vi "StartClone.vi"(7 "ShowPanel? (f)":bool, 8 "error in (no error)":errorcluster, 10 "ModuleName":string="unnamed", 11 "VI Refnum":refnum<vi>) -> (0 "error out":errorcluster, 1 "clBroadcastEvents":T1, 2 "VI Ref":refnum<vi>, 3 "ModuleAdmin":refnum<class "ModuleAdmin.lvclass">)   [LabVIEW 2018, in "FgenShared.lvlib"]
uses:
  FgenShared/FgenShared.lvlib
  FgenShared/clBroadcastEvents.ctl
  FgenShared/clEventType.ctl
  <userlib>/NIST/ModuleAdminLib/ModuleAdmin/ModuleAdmin.lvclass
  C:/Program Files (x86)/National Instruments/LabVIEW 2018/user.lib/NIST/ModuleAdminLib/ModuleAdminBase/ModuleAdminBase.lvclass
  <userlib>/NIST/ModuleAdminLib/CloneRegistration/CloneRegistration.lvclass
  <userlib>/NIST/ModuleAdminLib/ModuleAdmin/ModuleAdmin.lvclass/ModuleAdmin.ctl
  <userlib>/NIST/ModuleAdminLib/ModuleAdmin/Accessors/Write CloneRegRef.vi
  <userlib>/NIST/ModuleAdminLib/ModuleAdmin/Accessors/Write ShowPanel_.vi
  <vilib>/Utility/error.llb/Error Cluster From Error Code.vi
  <vilib>/ErrorRing/Error Ring.xnode
  <userlib>/NIST/ModuleAdminLib/ModuleAdminBase/ModuleAdminBase.lvclass
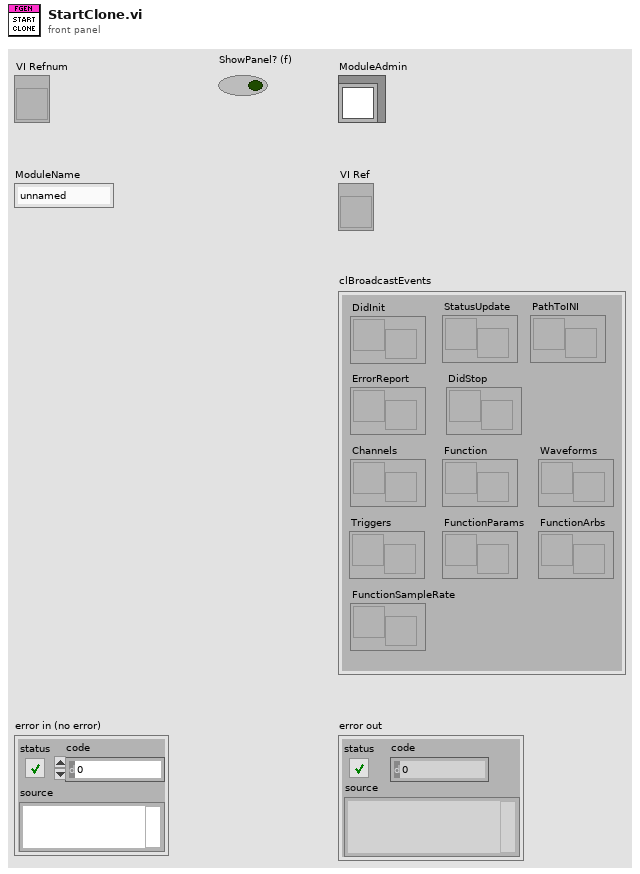
[diagram p1: front panel]
types:
  T1 = typedef "FgenShared.lvlib/clBroadcastEvents.ctl" = cluster{"DidInit":refnum<user-event>, "StatusUpdate":refnum<user-event>, "ErrorReport":refnum<user-event>, "DidStop":refnum<user-event>, "PathToINI":refnum<user-event>, "Channels":refnum<user-event>, "Function":refnum<user-event>, "Waveforms":refnum<user-event>, "Triggers":refnum<user-event>, "FunctionParams":refnum<user-event>, "FunctionArbs":refnum<user-event>, "FunctionSampleRate":refnum<user-event>}
  T2 = enum32{"Bad", "Idle", "Run top level", "Running"}
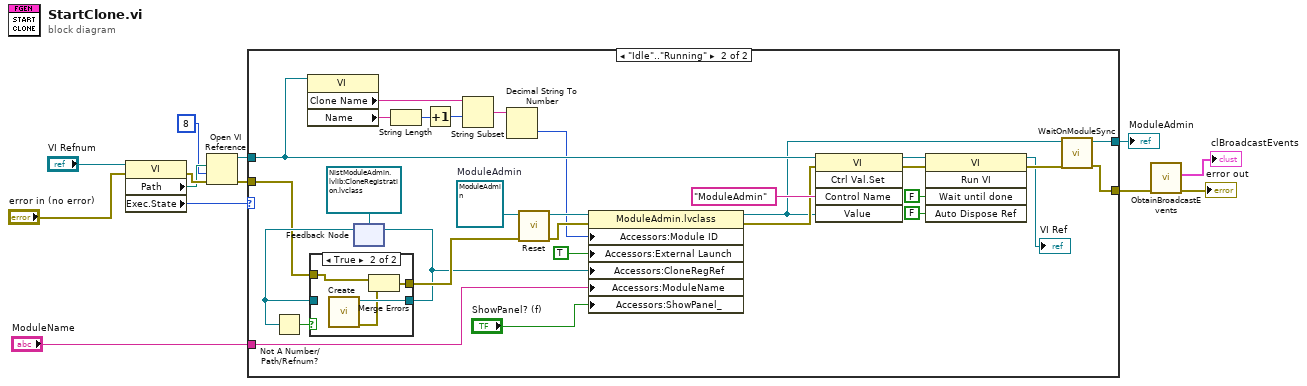
[diagram p0: block diagram]
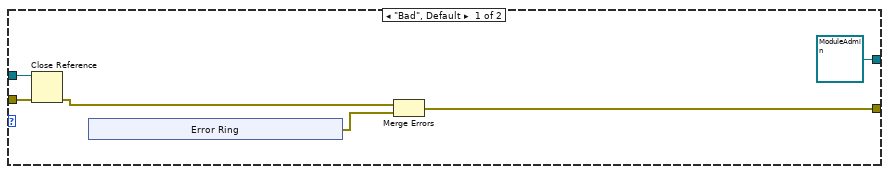
[diagram p2: hidden frame]
diagram:
  n1 = property class="VI"(reference="VI Refnum", error in="error in (no error)") -> (error out=w11:errorcluster, "Path"=w10:path, "Exec.State"=w12:T2)  [unwired: 1 out]
  n2 = Open VI Reference(vi path=w10, options=8, error in (no error)=w11) -> (vi reference=w8:refnum<vi>, error out=w9:errorcluster)  [unwired: 3 in]
  n3 = case shown="\"Idle\"..\"Running\"" w12 {
    tunnel: w9 -> [w19 w29]
    tunnel: w8 -> [w18 w44]
    tunnel: [w15 w34] -> w5
    tunnel: "ModuleName" -> [_ w33]
    tunnel: [refnum<class "ModuleAdmin.lvclass"> refnum ("ModuleAdmin") w26] -> w1
    frame "Bad", Default {
      n4 = Close Reference(reference=w18, error in (no error)=w19) -> (error out=w17:errorcluster)
      n5 = xnode "Error Ring"() -> ("error out"=w16:errorcluster)
      n6 = Merge Errors(w17, w16) -> (w15:errorcluster)
    }
    frame "Idle".."Running" {
      w48 = refnum<class "ModuleAdmin.lvclass"> refnum  # ModuleAdmin
      n7 = property class="VI"(reference=w44) -> ("Clone Name"=w50:string, "Name"=w53:string)  [unwired: 1 in, 2 out]
      n8 = feedback #1(refnum<data-value> refnum ("CloneRegRef")) -> (w32:refnum<data-value>)
      n9 = Not A Number/Path/Refnum?(number/path/refnum=w32) -> (NaN/Path/Refnum?=w31:bool)
      n10 = case shown="True" w31 {
        tunnel: [w55 w59] -> w27
        tunnel: w32 -> [w55 _]
        tunnel: w29 -> [w54 w57]
        tunnel: [w54 w56] -> w28
        frame False {
        }
        frame True {
          n11 = call <userlib>:"Create.vi"() -> ("error out"=w58:errorcluster, "CloneRegRef"=w59:refnum<data-value>)  [unwired: 10 in]
          n12 = Merge Errors(w57, w58) -> (w56:errorcluster)
        }
      }
      n13 = feedback-in #1(w27) -> ()
      n14 = String Length(string=w53) -> (length=w52:i32)
      n15 = Increment(x=w52) -> (x+1=w51:i32)
      n16 = String Subset(string=w50, offset (0)=w51) -> (substring=w49:string)  [unwired: 1 in]
      n17 = Decimal String To Number(string=w49) -> (number=w36:i32)  [unwired: 2 in, 1 out]
      n18 = call <userlib>:"Reset.vi"("error in (no error)"=w28, "Mod Admin in"=w48) -> ("error out"=w47:errorcluster, "Mod Admin out"=w46:refnum<class "ModuleAdmin.lvclass">)  [unwired: 8 in]
      n19 = property class="ModuleAdmin.lvclass"(reference=w46, error in=w47, "Accessors:Module ID"=w36, "Accessors:External Launch"=TRUE ("External Launch"), "Accessors:CloneRegRef"=w27, "Accessors:ModuleName"=w33, "Accessors:ShowPanel_"="ShowPanel? (f)") -> (reference out=w35:refnum<class "ModuleAdmin.lvclass">, error out=w37:errorcluster)
      n20 = invoke class="VI" method="Ctrl Val.Set"(reference=w44, error in=w37, "Control Name"="ModuleAdmin", "Value"=w35) -> (reference out=w42:refnum<vi>, error out=w41:errorcluster)  [unwired: 1 in, 3 out]
      n21 = invoke class="VI" method="Run VI"(reference=w42, error in=w41, "Wait until done"=FALSE ("Wait Until Done"), "Auto Dispose Ref"=FALSE ("Auto Dispose Reference")) -> (reference out=→"VI Ref":refnum<vi>, error out=w38:errorcluster)  [unwired: 1 in, 3 out]
      n22 = call <userlib>:"WaitOnModuleSync.vi"("error in (no error)"=w38, "ModuleAdmin"=w35) -> ("error out"=w34:errorcluster, "ModuleAdmin"=w26:refnum<class "ModuleAdmin.lvclass">)  [unwired: 8 in]
    }
  }
  "ModuleAdmin" <- w1
  n23 = call "ObtainBroadcastEvents.vi"("error in (no error)"=w5) -> ("error out"=→"error out":errorcluster, "FgenBroadcastEvents"=→"clBroadcastEvents":T1)  [unwired: 9 in]
